vi "Practica 4 - Cociente y Residuo.vi"() -> ()   [LabVIEW 2023]
panel:
  out "COCIENTE":dbl
  out "RESIDUO":dbl
  in  "DIVIDENDO":dbl
  in  "DIVISOR":dbl
  # "Cociente y Residuo"
  # "Operacion"
  # "Resultado"
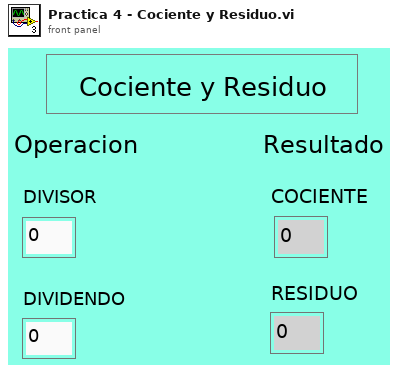
[diagram p1: front panel]
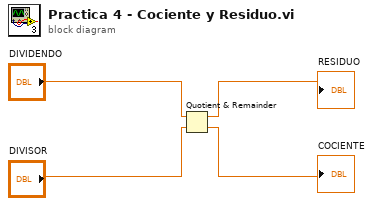
[diagram p0: block diagram]
diagram:
  n1 = Quotient & Remainder(x="DIVIDENDO", y="DIVISOR") -> (x-y*floor(x/y)=→"RESIDUO":dbl, floor(x/y)=→"COCIENTE":dbl)
